vi "MLE.vi"(1 "input range":cluster{"x0":dbl, "x1":dbl} {"x1" format="%.2f"; "x0" format="%.2f"}, 2 "channel width (ns)":dbl format="%.2f", 3 "lifetime histograms":u32[](array[numeric])) -> (0 "lifetime (ns)":dbl[](array[numeric]) format="%.2f")   [LabVIEW 2009]
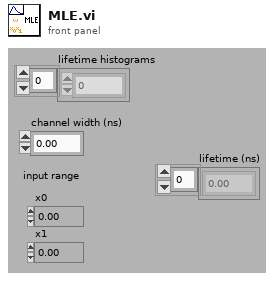
[diagram p1: front panel]
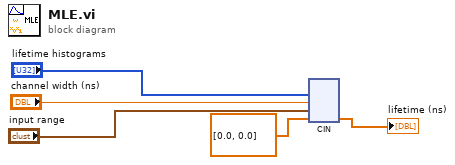
[diagram p0: block diagram]
diagram:
  n1 = cin("lifetime histograms", "channel width (ns)", "input range", dbl[] [0.0, 0.0] ("input")) -> (→"lifetime (ns)":dbl[])  [unwired: 3 in]
